vi "1 equals 2.vi"() -> ()   [LabVIEW 2025]
uses:
  <vilib>/Analysis/2dsp.llb/Real FFT.vi
  <vilib>/Analysis/NI_AALBase.lvlib
  <vilib>/Analysis/NI_AALPro.lvlib
panel:
  out "The Signal":dbl[](graph)
  out "The Spectrum":dbl[](graph)
  out "The Signal (Zoom In)":dbl[](graph)
  out "The Spectrum (Zoom In)":dbl[][](graph)
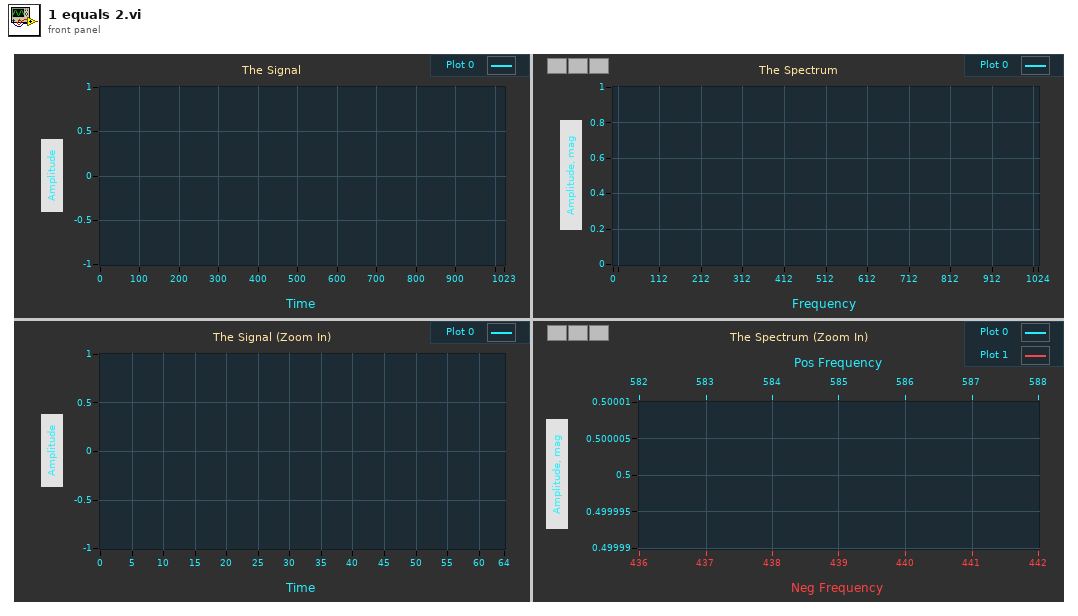
[diagram p1: front panel]
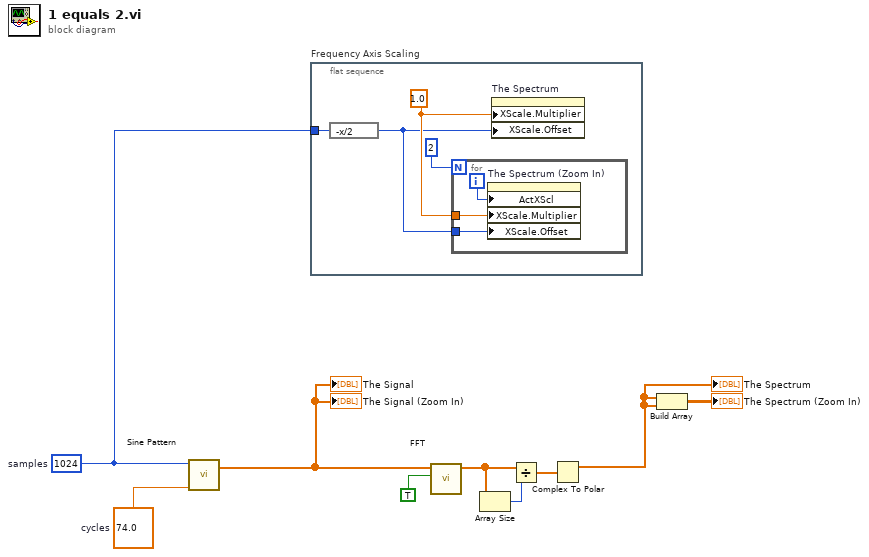
[diagram p0: block diagram]
diagram:
  w8 = 74.0  # cycles
  w7 = 1024  # samples
  n1 = call <vilib>:"Sine Pattern.vi"("cycles"=w8, "samples"=w7) -> ("Sinusoidal Pattern"=w1:dbl[])  [unwired: 2 in, 1 out]
  "The Signal" <- w1
  "The Signal (Zoom In)" <- w1
  n2 = flat-sequence "Frequency Axis Scaling" {
    tunnel: w7 -> [w13]
    frame #0 {
      w12 = 1.0 ("X Scale.Offset and Multiplier:Multiplier")
      n3 = expression code="-x/2"(w13) -> (w11:i32)
      n4 = for {
        N: 2 -> [_]
        tunnel: w12 -> [w16]
        tunnel: w11 -> [w15]
        i -> [w14]
        n5 = property on="The Spectrum (Zoom In)" class="WFGraph (strict)"("ActXScl"=w14, "XScale.Multiplier"=w16, "XScale.Offset"=w15) -> ()  [unwired: 2 in, 2 out]
      }
      n6 = property on="The Spectrum" class="WFGraph (strict)"("XScale.Multiplier"=w12, "XScale.Offset"=w11) -> ()  [unwired: 2 in, 2 out]
    }
  }
  n7 = call-poly <vilib>:"FFT.vi"("shift?"=TRUE, "X"=w1) -> ("FFT {X}"=w6:cdb[])  [unwired: 8 in, 1 out]
  n8 = Array Size(array=w6) -> (size(s)=w5:i32)
  n9 = Divide(x=w6, y=w5) -> (x/y=w4:cdb[])
  n10 = Complex To Polar(r * e^(i*theta)=w4) -> (r=w2:dbl[])  [unwired: 1 out]
  "The Spectrum" <- w2
  n11 = Build Array(w2, w2) -> (→"The Spectrum (Zoom In)":dbl[][])
